vi "Array Reduced Mean & SDV.vi"(9 "standard deviation":dbl, 10 "mean":dbl, 11 "Array":dbl[](array[numeric])) -> (1 "Reduced Standard Deviation":dbl, 2 "Reduced Array mean":dbl, 3 "Reduced Array":dbl[](array[numeric]))   [LabVIEW 2021, in "Math.lvlib"]
doc: "Computes the <B>Reduced Mean</B> and <B>Reduced Standard Deviation</B> of an <B>Array</B> by limiting the analysis to the \"peak\" part of the array, i.e. for points within [m - SDV, m +SDV], where m is the array <B>mean</B> and <B>standard deviation</B>."
uses:
  7da2e921-b6d2-4606-b168-572b6321dc80.vi
  <vilib>/Comparison/Less/Less Functor/Less Functor.lvclass
  Math.lvlib
  <vilib>/Analysis/NI_AALBase.lvlib
panel:
  # "see the AlliGator License on the block diagram (Ctrl+E or Window:Show Block Diagram)"
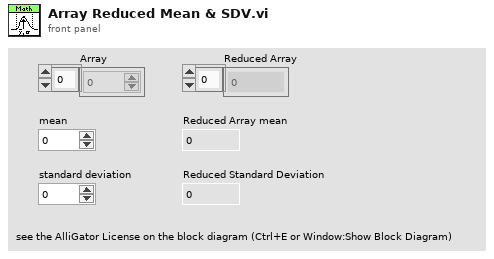
[diagram p1: front panel]
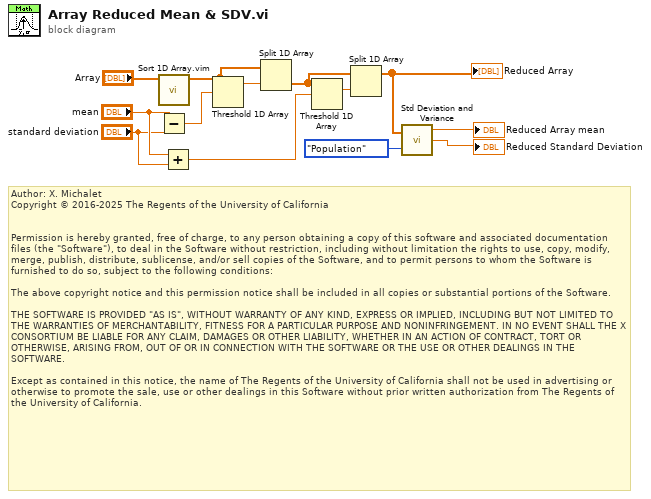
[diagram p0: block diagram]
diagram:
  # "Author: X. Michalet\nCopyright © 2016-2025 The Regents of the University of California\n \n\nPermission is hereby granted, free of charge, to any person obtaining a copy of this software and associated documentation files (the \"Software\"), to deal in the Software without restriction, including without limitation the rights to use, copy, modify, merge, publish, distribute, sublicense, and/or sell copies of the Software, and to permit persons to whom the Software is furnished to do so, subject to the following conditions:\n\nThe above copyright notice and this permission notice shall be included in all copies or substantial portions of the Software.\n\nTHE SOFTWARE IS PROVIDED \"AS IS\", WITHOUT WARRANTY OF ANY KIND, EXPRESS OR IMPLIED, INCLUDING BUT NOT LIMITED TO THE WARRANTIES OF MERCHANTABILITY, FITNESS FOR A PARTICULAR PURPOSE AND NONINFRINGEMENT. IN NO EVENT SHALL THE X CONSORTIUM BE LIABLE FOR ANY CLAIM, DAMAGES OR OTHER LIABILITY, WHETHER IN AN ACTION OF CONTRACT, TORT OR OTHERWISE, ARISING FROM, OUT OF OR IN CONNECTION WITH THE SOFTWARE OR THE USE OR OTHER DEALINGS IN THE SOFTWARE.\n\nExcept as contained in this notice, the name of The Regents of the University of California shall not be used in advertising or otherwise to promote the sale, use or other dealings in this Software without prior written authorization from The Regents of the University of California."
  n1 = call "Sort 1D Array.vim"("unsorted array"="Array") -> ("sorted array"=w1:dbl[])  [unwired: 10 in]
  n2 = Subtract(x="mean", y="standard deviation") -> (x-y=w13:dbl)
  n3 = Add(x="mean", y="standard deviation") -> (x+y=w8:dbl)
  n4 = Threshold 1D Array(2:w13, 3:w1) -> (0:w12:dbl)  [unwired: 1 in]
  n5 = Split 1D Array(array=w1, index=w12) -> (second subarray=w6:dbl[])  [unwired: 1 out]
  n6 = Threshold 1D Array(2:w8, 3:w6) -> (0:w7:dbl)  [unwired: 1 in]
  n7 = Split 1D Array(array=w6, index=w7) -> (first subarray=w5:dbl[])  [unwired: 1 out]
  "Reduced Array" <- w5
  n8 = call <vilib>:"Std Deviation and Variance.vi"("X"=w5, "Weighting (Sample)"=enum16{"Sample", "Population"}."Population") -> ("mean"=→"Reduced Array mean":dbl, "standard deviation"=→"Reduced Standard Deviation":dbl)  [unwired: 1 out]
